vi "Handle.vi"(7 "Queue Actor in":refnum<class "Queue Actor.lvclass">, 11 "Error Queue State in":refnum<class "Error Queue State.lvclass">) -> (2 "Destroy?":bool, 5 "Queue Actor out":refnum<class "Queue Actor.lvclass">)   [LabVIEW 2021, in "jettl.lvlib" / "Error Queue State.lvclass"]
uses:
  Error Queue State.lvclass
  Queue Actor/Queue Actor.lvclass
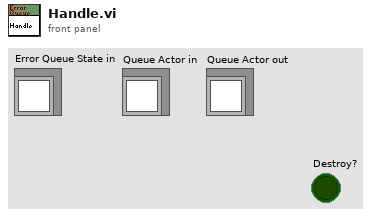
[diagram p1: front panel]
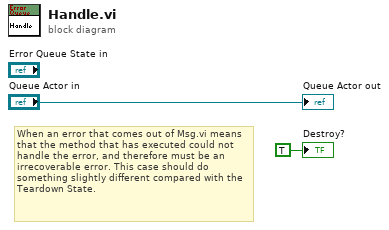
[diagram p0: block diagram]
diagram:
  # "When an error that comes out of Msg.vi means that the method that has executed could not handle the error, and therefore must be an irrecoverable error. This case should do something slightly different compared with the Teardown State."
  "Destroy?" <- TRUE ("Destroy?")
  "Queue Actor out" <- "Queue Actor in"
